vi "dfd_Maxflat Filter Design Find Table.vi"(7 "symmetric FIR ? (T)":bool, 10 "denominator order":i32=2, 11 "numerator order":i32=2) -> (3 "table":dbl[](array[numeric]))   [LabVIEW 2017, in "NI_DigFilter_Design.lvlib"]
doc: "Builds the table to keep the <B>L</B>, <B>M</B>, <B>N</B>, 0.5*min (angle frequency) and 0.5*mix (angle frequency) ."
uses:
  <vilib>/addons/Digital Filter Design/NI_DigFilter_Design.lvlib
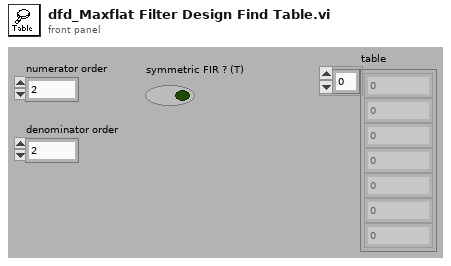
[diagram p1: front panel]
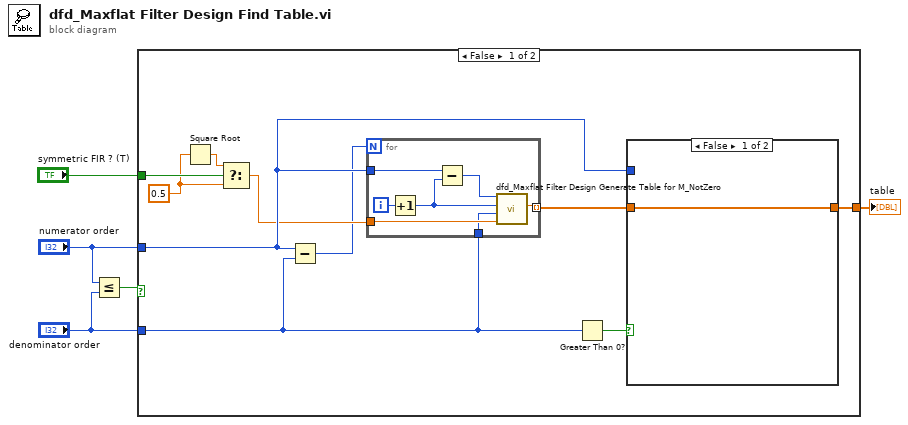
[diagram p0: block diagram]
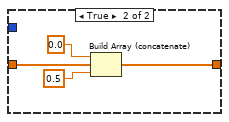
[diagram p2: hidden frame]
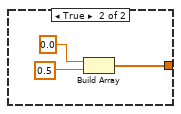
[diagram p3: hidden frame]
diagram:
  n1 = Less Or Equal?(x="numerator order", y="denominator order") -> (x <= y?=w5:bool)
  n2 = case shown="False" w5 {
    tunnel: "numerator order" -> [w8 _]
    tunnel: "denominator order" -> [w15 _]
    tunnel: "symmetric FIR ? (T)" -> [w12 _]
    tunnel: [w14 w28] -> w1
    frame False {
      w10 = 0.5
      n3 = Square Root(x=w10) -> (sqrt(x)=w11:dbl)
      n4 = Select(t=w11, s=w12, f=w10) -> (s? t:f=w7:dbl)
      n5 = Subtract(x=w8, y=w15) -> (x-y=w6:i32)
      n6 = for {
        N: w6 -> [_]
        tunnel: w8 -> [w27]
        tunnel: w15 -> [w25]
        tunnel: w7 -> [w26]
        tunnel: [w23] -> w13 mode=indexing
        i -> [w22]
        n7 = Increment(x=w22) -> (x+1=w21:i32)
        n8 = Subtract(x=w27, y=w21) -> (x-y=w24:i32)
        n9 = call <vilib>:"dfd_Maxflat Filter Design Generate Table for M_NotZero.vi"("H0"=w26, "N"=w25, "M"=w21, "L"=w24) -> ("fc"=w23:dbl)  [unwired: 7 out]
      }
      n10 = Greater Than 0?(x=w15) -> (x > 0?=w9:bool)
      n11 = case shown="False" w9 {
        tunnel: w13 -> [w16 w20]
        tunnel: [w16 w17] -> w14
        tunnel: w8 -> [_ _]
        frame False {
        }
        frame True {
          n12 = Build Array (concatenate)(0.0 ("element"), w20, 0.5 ("element")) -> (w17:dbl[])
        }
      }
    }
    frame True {
      n13 = Build Array(0.0 ("element"), 0.5 ("element")) -> (w28:dbl[])
    }
  }
  "table" <- w1
